vi "getDforce.vi"(6 "ForceDesired":dbl, 7 "Desired Direction":dbl[](array[numeric])) -> (3 "FX FY 0 0 0 0":dbl[](array[numeric]))   [LabVIEW 2017]
uses:
  <vilib>/Analysis/_algsub.llb/Real Vector Norm.vi
  <vilib>/Analysis/NI_AALPro.lvlib
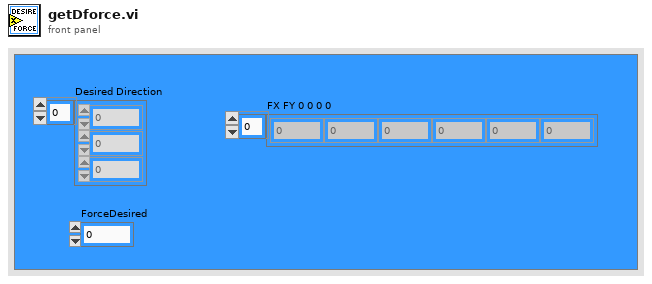
[diagram p1: front panel]
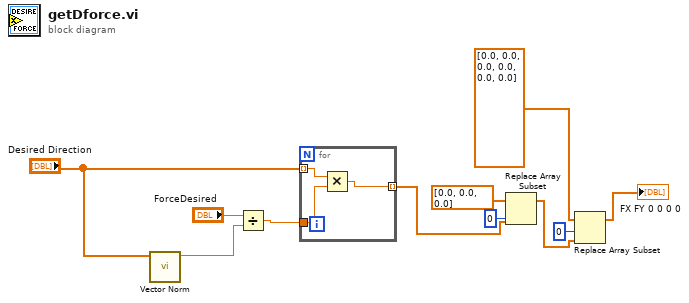
[diagram p0: block diagram]
diagram:
  n1 = call-poly <vilib>:"Vector Norm.vi"("Input Vector"="Desired Direction") -> ("norm"=w2:dbl)  [unwired: 9 in, 1 out]
  n2 = Divide(x="ForceDesired", y=w2) -> (x/y=w10:dbl)
  n3 = for {
    tunnel: "Desired Direction" -> [w14] mode=indexing
    tunnel: w10 -> [w13]
    tunnel: [w12] -> w7 mode=indexing
    n4 = Multiply(x=w14, y=w13) -> (x*y=w12:dbl)
  }
  n5 = Replace Array Subset(array=dbl[] [0.0, 0.0, 0.0], new element=w7, index=0) -> (w4:dbl[])
  n6 = Replace Array Subset(array=dbl[] [0.0, 0.0, 0.0, 0.0, 0.0, 0.0] ("element"), new element=w4, index=0) -> (→"FX FY 0 0 0 0":dbl[])
